vi "State_Machine.vi"(8 "error in (no error)":errorcluster caption="entrée d'erreur (pas d'erreur)", 11 "Flash_AVRDUDE en entrée":refnum<class "Flash_P2056.lvclass">) -> (0 "error out":errorcluster caption="sortie d'erreur", 2 "Json_String":string, 3 "Flash_AVRDUDE en sortie":refnum<class "Flash_P2056.lvclass">)   [LabVIEW 2020, in "Library Test.lvlib" / "Flash_P2056.lvclass"]
uses:
  Flash_P2056.lvclass
  C:/Users/ngarcin/OneDrive - Altyor/Standard TB/Class/Test/Test (Default)/Test (Default).lvclass
  Flash_P2056.lvclass/Flash_P2056.ctl
panel:
  out "String In progress":string
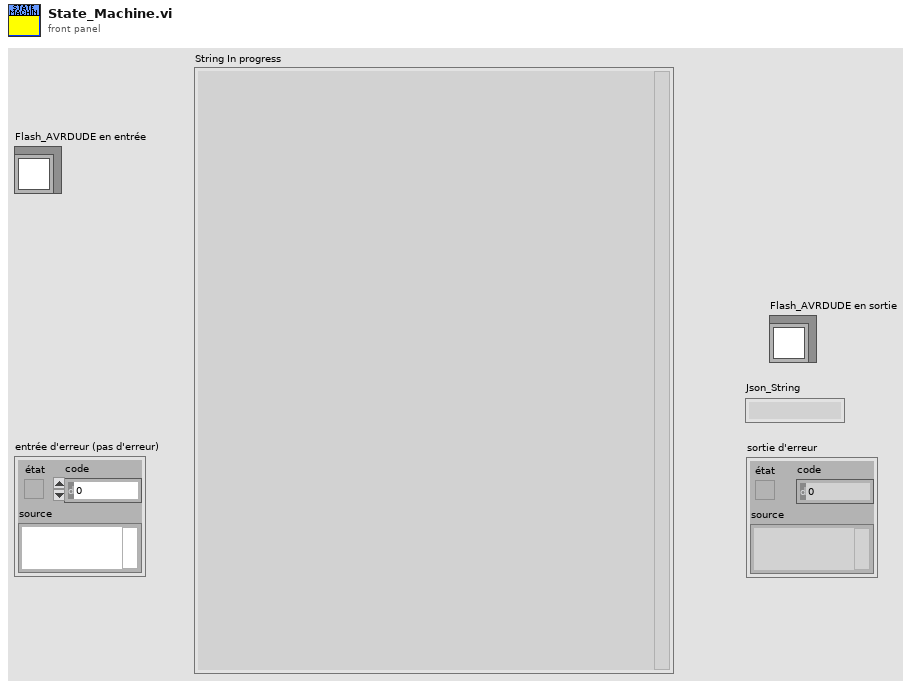
[diagram p1: front panel]
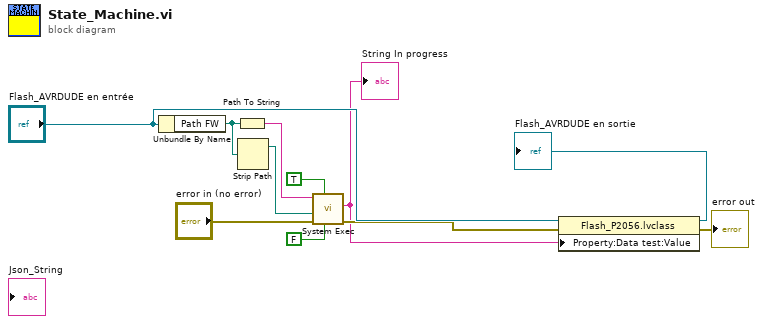
[diagram p0: block diagram]
diagram:
  n1 = Unbundle By Name("Flash_AVRDUDE en entrée") -> ("Path FW"=w3:path)
  n2 = Path To String(path=w3) -> (string=w4:string)
  n3 = Strip Path(path=w3) -> (stripped path=w2:path)  [unwired: 1 out]
  n4 = call <vilib>:"System Exec.vi"("run minimized? (F)"=FALSE, "wait until completion? (T)"=TRUE, "error in (no error)"="error in (no error)", "working directory"=w2, "command line"=w4) -> ("error out"=w5:errorcluster, "standard error"=w1:string)  [unwired: 3 in, 2 out]
  "String In progress" <- w1
  n5 = property class="Flash_P2056.lvclass"(reference="Flash_AVRDUDE en entrée", error in=w5, "Property:Data test:Value"=w1) -> (reference out=→"Flash_AVRDUDE en sortie":refnum<class "Flash_P2056.lvclass">, error out=→"error out":errorcluster)
